vi "Unregister API.vi"(8 "error in (no error)":errorcluster, 10 "API":refnum<class "API.lvclass">, 11 "VolatusAPI in":refnum<class "VolatusAPI.lvclass">) -> (0 "error out":errorcluster, 3 "VolatusAPI out":refnum<class "VolatusAPI.lvclass">)   [LabVIEW 2020, in "Volatus.lvlib" / "VolatusAPI.lvclass"]
uses:
  VolatusAPI.lvclass
  VolatusAPI.lvclass/VolatusAPI.ctl
  Identity/Identity.lvclass
  API/API.lvclass
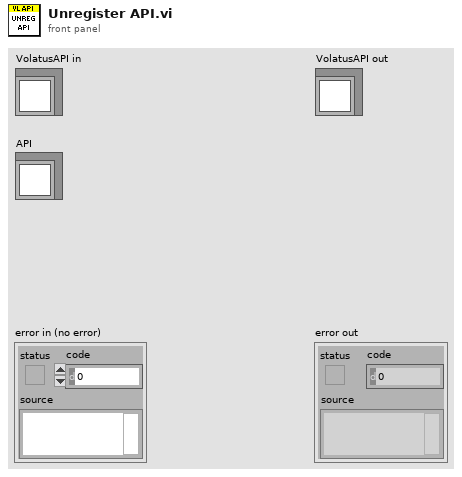
[diagram p1: front panel]
types:
  T1 = typedef "Volatus.lvlib/VolatusAPI.lvclass/APIs Ref.ctl" = cluster{"API Numbers":map{string, u32}, "APIs":map{u32, refnum<class "API.lvclass">}, "Next API":u32}
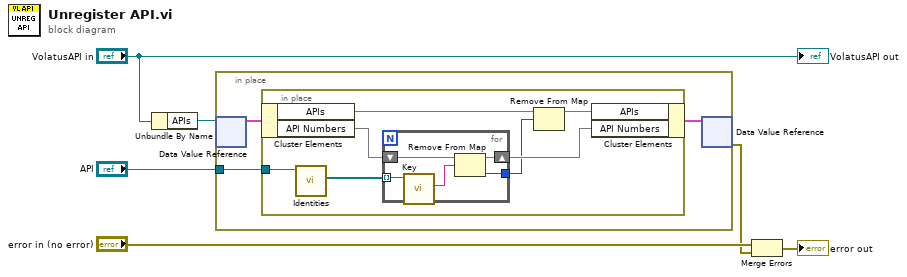
[diagram p0: block diagram]
diagram:
  n1 = Unbundle By Name("VolatusAPI in") -> ("APIs"=w3:refnum<data-value>)
  n2 = in-place {
    in-place-border: "API" -> [w9]
    n3 = in-place-dvr #1(w3) -> (w8:T1)  [unwired: 1 out]
    n4 = in-place {
      in-place-border: w9 -> [w16]
      n5 = in-place-cluster #2(w8) -> ("APIs"=w12:map{u32, refnum<class "API.lvclass">}, "API Numbers"=w14:map{string, u32})
      n6 = call-dynamic "Identities.vi"("API in"=w16) -> ("Identities"=w15:refnum<class "Identity.lvclass">[])  [unwired: 8 in, 2 out]
      n7 = for {
        tunnel: w15 -> [w21] mode=indexing
        shift-right: [w18] -> w13
        shift-left: w14 -> [w20]
        tunnel: [w17] -> w10
        n8 = call "Key.vi"("Identity in"=w21) -> ("Key"=w19:string)  [unwired: 10 in]
        n9 = Remove From Map(10:w19, 11:w20) -> (1:w17:u32, 3:w18:map{string, u32})  [unwired: 1 out]
      }
      n10 = Remove From Map(10:w10, 11:w12) -> (3:w11:map{u32, refnum<class "API.lvclass">})  [unwired: 2 out]
      n11 = in-place-cluster #2("APIs"=w11, "API Numbers"=w13) -> (w7:T1)
    }
    n12 = in-place-dvr #1(w7) -> (w1:errorcluster)  [unwired: 1 out]
  }
  n13 = Merge Errors("error in (no error)", w1) -> (→"error out":errorcluster)
  "VolatusAPI out" <- "VolatusAPI in"
